vi "Graphe.vi"(8 "Error in (no error)":errorcluster, 10 "number":i32, 11 "Connection In":refnum<k7>) -> (0 "Error out":errorcluster, 2 "Graphe de temperature":cluster{timestamp[], dbl[]}(graph) caption="XY Graph - Dark", 3 "graphe de pression":cluster{timestamp[], dbl[]}(graph) caption="XY Graph - Dark", 5 "Connection Out":refnum<k7>)   [LabVIEW 2019]
panel:
  out "error out":errorcluster
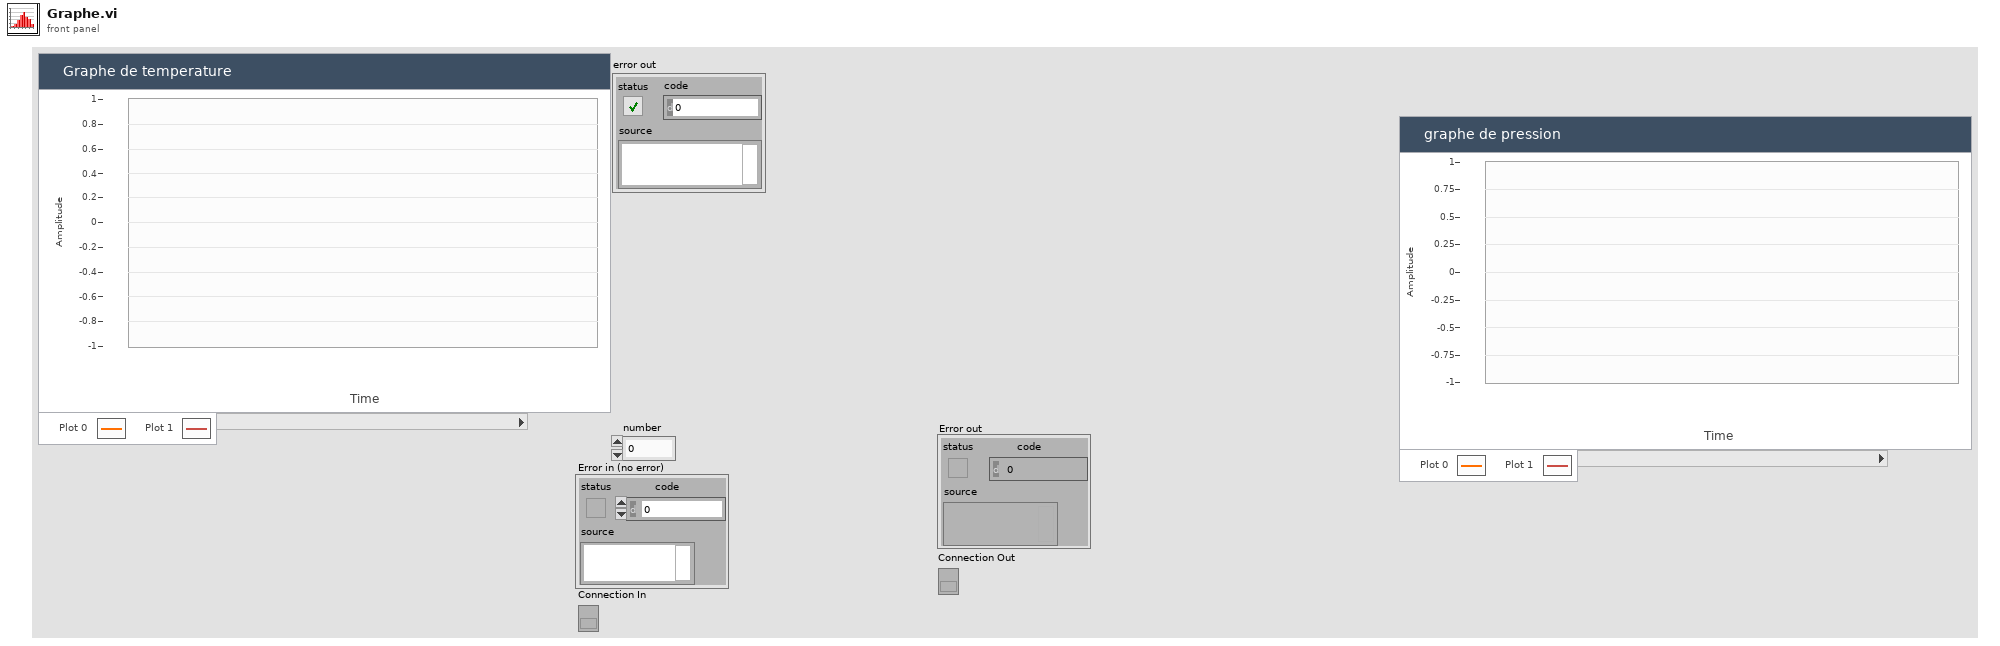
[diagram p1: front panel]
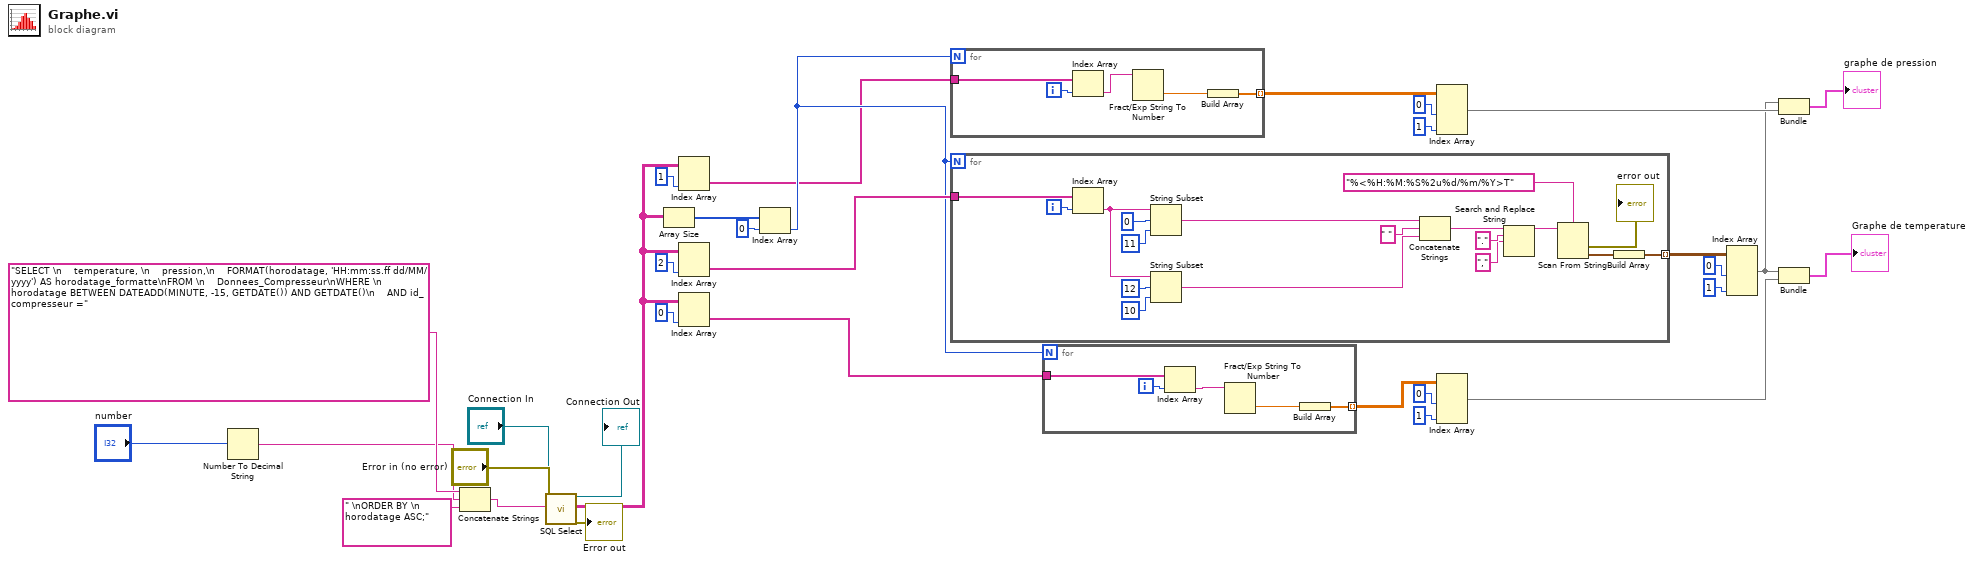
[diagram p0: block diagram]
diagram:
  n1 = Number To Decimal String(number="number") -> (decimal integer string=w7:string)  [unwired: 1 in]
  n2 = Concatenate Strings("SELECT \n    temperature, \n    pression,\n    FORMAT(horodatage, 'HH:mm:ss.ff dd/MM/yyyy') AS horodatage_formatte\nFROM \n    Donnees_Compresseur\nWHERE \n    horodatage BETWEEN DATEADD(MINUTE, -15, GETDATE()) AND GETDATE()\n    AND id_compresseur =" ("SQL Query"), w7, " \nORDER BY \n    horodatage ASC;" ("string")) -> (w5:string)
  n3 = call <vilib>:"SQL Select.vi"("Connection In"="Connection In", "SQL Query"=w5, "Error in (no error)"="Error in (no error)") -> ("Connection Out"=→"Connection Out":refnum<k7>, "Data"=w10:string[][], "Error out"=→"Error out":errorcluster)  [unwired: 14 in]
  n4 = Array Size(array=w10) -> (size(s)=w32:i32[])
  n5 = Index Array(array=w10, index (col)=1 ("disabled index (col)")) -> (element=w17:string[])  [unwired: 1 in]
  n6 = Index Array(array=w10, index (col)=2 ("disabled index (col)")) -> (element=w28:string[])  [unwired: 1 in]
  n7 = Index Array(array=w10, index (col)=0 ("disabled index (col)")) -> (element=w29:string[])  [unwired: 1 in]
  n8 = Index Array(array=w32, index=0) -> (element=w19:i32)
  n9 = for {
    N: w19 -> [_]
    tunnel: w17 -> [w36]
    tunnel: [w35] -> w14 mode=indexing
    i -> [w34]
    n10 = Index Array(array=w36, index=w34) -> (element=w38:string)
    n11 = Fract/Exp String To Number(string=w38) -> (number=w37:dbl)  [unwired: 3 in, 1 out]
    n12 = Build Array(w37) -> (w35:dbl[])
  }
  n13 = for {
    N: w19 -> [_]
    tunnel: w28 -> [w54]
    tunnel: [w52] -> w22 mode=indexing
    i -> [w55]
    n14 = Index Array(array=w54, index=w55) -> (element=w49:string)
    n15 = String Subset(string=w49, offset (0)=0, length (rest)=11 ("length (rest)")) -> (substring=w46:string)
    n16 = String Subset(string=w49, offset (0)=12, length (rest)=10 ("length (rest)")) -> (substring=w44:string)
    n17 = Concatenate Strings(w46, " " ("string"), w44) -> (w43:string)
    n18 = Search and Replace String(input string=w43, search string=".", replace string="," ("replace string (\"\")")) -> (result string=w40:string)  [unwired: 5 in, 3 out]
    n19 = Scan From String(format string="%<%H:%M:%S%2u%d/%m/%Y>T", input string=w40) -> (error out=→"error out":errorcluster, output 1=w53:timestamp)  [unwired: 3 in, 2 out]
    n20 = Build Array(w53) -> (w52:timestamp[])
  }
  n21 = for {
    N: w19 -> [_]
    tunnel: w29 -> [w60]
    tunnel: [w57] -> w25 mode=indexing
    i -> [w61]
    n22 = Index Array(array=w60, index=w61) -> (element=w59:string)
    n23 = Fract/Exp String To Number(string=w59) -> (number=w58:dbl)  [unwired: 3 in, 1 out]
    n24 = Build Array(w58) -> (w57:dbl[])
  }
  n25 = Index Array(array=w14, index (col) #1=0 ("disabled index (col)"), index (col) #2=1 ("index (col)")) -> (element #1=w13:dbl[])  [unwired: 2 in, 1 out]
  n26 = Index Array(array=w25, index (col) #1=0 ("disabled index (col)"), index (col) #2=1 ("index (col)")) -> (element #1=w21:dbl[])  [unwired: 2 in, 1 out]
  n27 = Index Array(array=w22, index (col) #1=0 ("disabled index (col)"), index (col) #2=1 ("index (col)")) -> (element #1=w12:timestamp[])  [unwired: 2 in, 1 out]
  n28 = Bundle(w12, w13) -> (→"graphe de pression":cluster{timestamp[], dbl[]})  [unwired: 1 in]
  n29 = Bundle(w12, w21) -> (→"Graphe de temperature":cluster{timestamp[], dbl[]})  [unwired: 1 in]
